vi "SimpleConsumer.vi"(8 "error in (no error)":errorcluster, 9 "Partition":i32, 10 "Topic":string="ExampleData1", 11 "Kafka Broker":string="getafix.ni.corp.natinst.com:9092") -> (0 "error out":errorcluster, 2 "Num Events":i64=-1, 3 "Events":T1[](array[typedef]))   [LabVIEW 2019]
uses:
  API/KafkaConsumerEvent.ctl
  API/LVKafka.lvlib
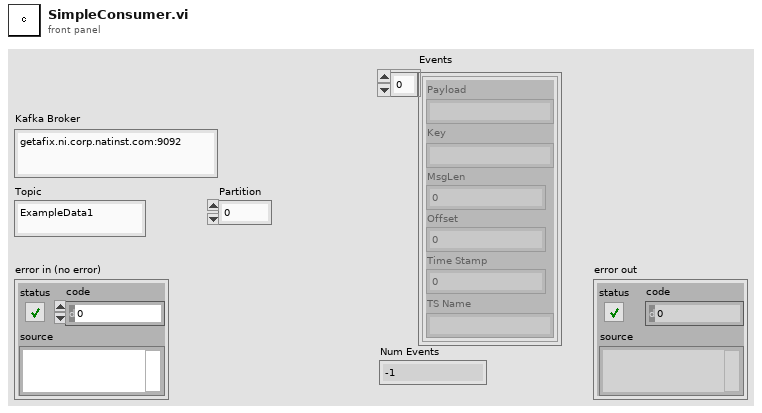
[diagram p1: front panel]
types:
  T1 = typedef "LVKafka.lvlib/KafkaConsumerEvent.ctl" = cluster{"Payload":string, "Key":string, "MsgLen":u64, "Offset":i64, "Time Stamp":i64, "TS Name":string}
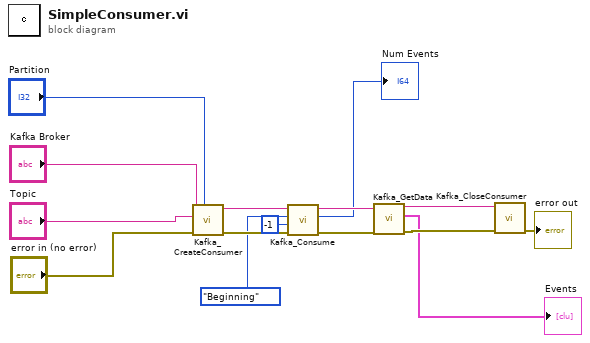
[diagram p0: block diagram]
diagram:
  n1 = call "Kafka_CreateConsumer.vi"("Partition"="Partition", "error in (no error)"="error in (no error)", "Topic"="Topic", "Kafka Broker"="Kafka Broker") -> ("error out"=w10:errorcluster, "Consumer Handle"=w9:string)  [unwired: 6 in]
  n2 = call "Kafka_Consume.vi"("error in (no error)"=w10, "Max Events"=i64 -1, "Kafka Offset"=enum16{"Beginning", "End", "Offset"}."Beginning", "Consumer Handle"=w9) -> ("error out"=w6:errorcluster, "Num Events"=→"Num Events":i64, "Consumer Handle"=w4:string)  [unwired: 4 in, 1 out]
  n3 = call "Kafka_GetData.vi"("error in (no error)"=w6, "Consumer Handle"=w4) -> ("error out"=w5:errorcluster, "Events"=→"Events":T1[], "Consumer Handle"=w3:string)  [unwired: 7 in]
  n4 = call "Kafka_CloseConsumer.vi"("error in (no error)"=w5, "Consumer Handle"=w3) -> ("error out"=→"error out":errorcluster)  [unwired: 8 in, 1 out]
